vi "check encoders.vi"(2 "Right (Y)":dbl, 3 "Left (X)":dbl) -> (0 "Right (Y) Out":dbl, 1 "Left (X) Out":dbl)   [LabVIEW 2013]
uses:
  typedefs/fg_typedef.ctl
  typedefs/Dashboard/drive safety.ctl
panel:
  # "Check encoder to make sure it is plugged in and working"
  # "tell status to dashboard"
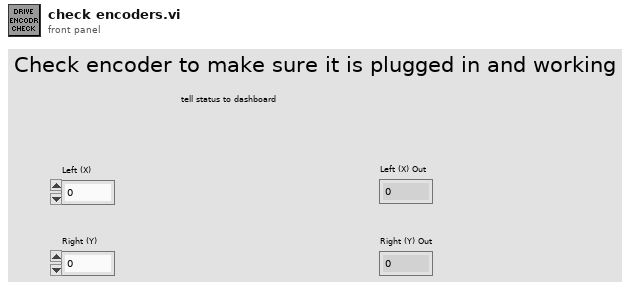
[diagram p1: front panel]
types:
  T1 = typedef "drive safety.ctl" = cluster{"Left - Encoder Failure":bool, "Left - No Rate Read":bool, "Right - Encoder Failure":bool, "Right - No Rate Read":bool}
  T2 = typedef "fg_typedef.ctl" = enum16{"Get", "Set"}
  T3 = typedef "WPI_EncoderDevRef.ctl" = cluster{"DevStatus":errorcluster, "EncoderIndex":T4, "CounterIndex":T5, "DistancePerCount":dbl, "Decoding Type":T6}
  T4 = typedef "FPGA_EncoderIdx.ctl" = enum8{"Enc 0", "Enc 1", "Enc 2", "Enc 3", "Invalid"}
  T5 = typedef "FPGA_CounterCtrSystemIndex.ctl" = enum8{"Ctr 0", "Ctr 1", "Ctr 2", "Ctr 3", "Ctr 4", "Ctr 5", "Ctr 6", "Ctr 7", "Invalid"}
  T6 = typedef "WPI_EncoderType.ctl" = enum16{"1x", "2x", "4x"}
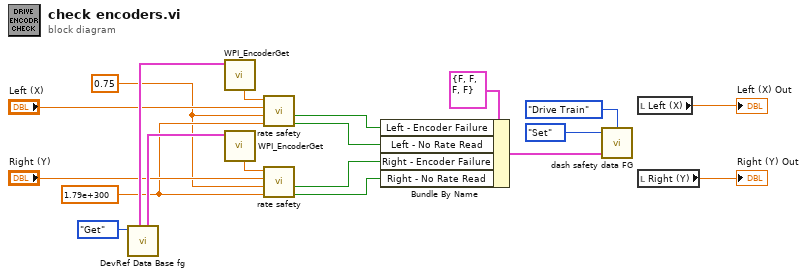
[diagram p0: block diagram]
diagram:
  w11 = 0.75 ("Cutoff Rate")
  w12 = 1.79e+300 ("Max Rate")
  n1 = call "DevRef Data Base fg.vi"("Menu"=fg_typedef."Get") -> ("right drive encoder"=w18:T3, "left drive encoder"=w19:T3)  [unwired: 2 in, 7 out]
  n2 = call <vilib>:"WPI_EncoderGet.vi"("EncoderDevRef"=w19) -> ("Rate"=w14:dbl)  [unwired: 5 in, 5 out]
  n3 = call <vilib>:"WPI_EncoderGet.vi"("EncoderDevRef"=w18) -> ("Rate"=w13:dbl)  [unwired: 5 in, 5 out]
  n4 = call "rate safety.vi"("Max Rate"=w12, "Cutoff Rate"=w11, "Desired Rate"="Left (X)", "Encoder Rate"=w14) -> ("No Rate Read"=w3:bool, "Encoder Failure"=w4:bool)  [unwired: 2 out]
  n5 = call "rate safety.vi"("Max Rate"=w12, "Cutoff Rate"=w11, "Desired Rate"="Right (Y)", "Encoder Rate"=w13) -> ("No Rate Read"=w1:bool, "Encoder Failure"=w2:bool)  [unwired: 2 out]
  n6 = Bundle By Name(cluster=T1 {"Left - Encoder Failure"=FALSE, "Left - No Rate Read"=FALSE, "Right - Encoder Failure"=FALSE, "Right - No Rate Read"=FALSE} ("Drive Safety Data"), "Left - Encoder Failure"=w4, "Left - No Rate Read"=w3, "Right - Encoder Failure"=w2, "Right - No Rate Read"=w1) -> (w5:T1)
  n7 = call "dash safety data FG.vi"("Mechanism"=enum16{"Arm", "Drive Train"}."Drive Train", "Drive Safety Data"=w5, "Menu"=fg_typedef."Set") -> ()  [unwired: 1 in, 2 out]
  n8 = local read "Left (X)"() -> (→"Left (X) Out":dbl)
  n9 = local read "Right (Y)"() -> (→"Right (Y) Out":dbl)
